vi "COBS_Unstuff.vi"(8 "error in (no error)":errorcluster, 11 "Suffed data":string) -> (0 "error out":errorcluster, 2 "Valid?":bool, 3 "Unstuffed String":string)   [LabVIEW 2015, in "Shore Library.lvlib"]
doc: "Unstuffs data stuffed with the COBS algorithm. This is used to take zeros out of a byte array to allow it to be used as a delimeter. \n\nhttps://en.wikipedia.org/wiki/Consistent_Overhead_Byte_Stuffing"
uses:
  Shore Library.lvlib
panel:
  out "unsigned byte array":u8[](array[numeric])
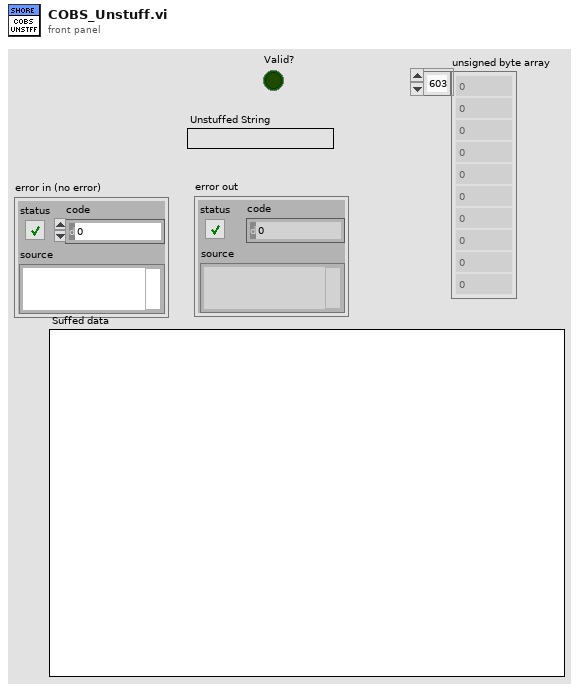
[diagram p1: front panel]
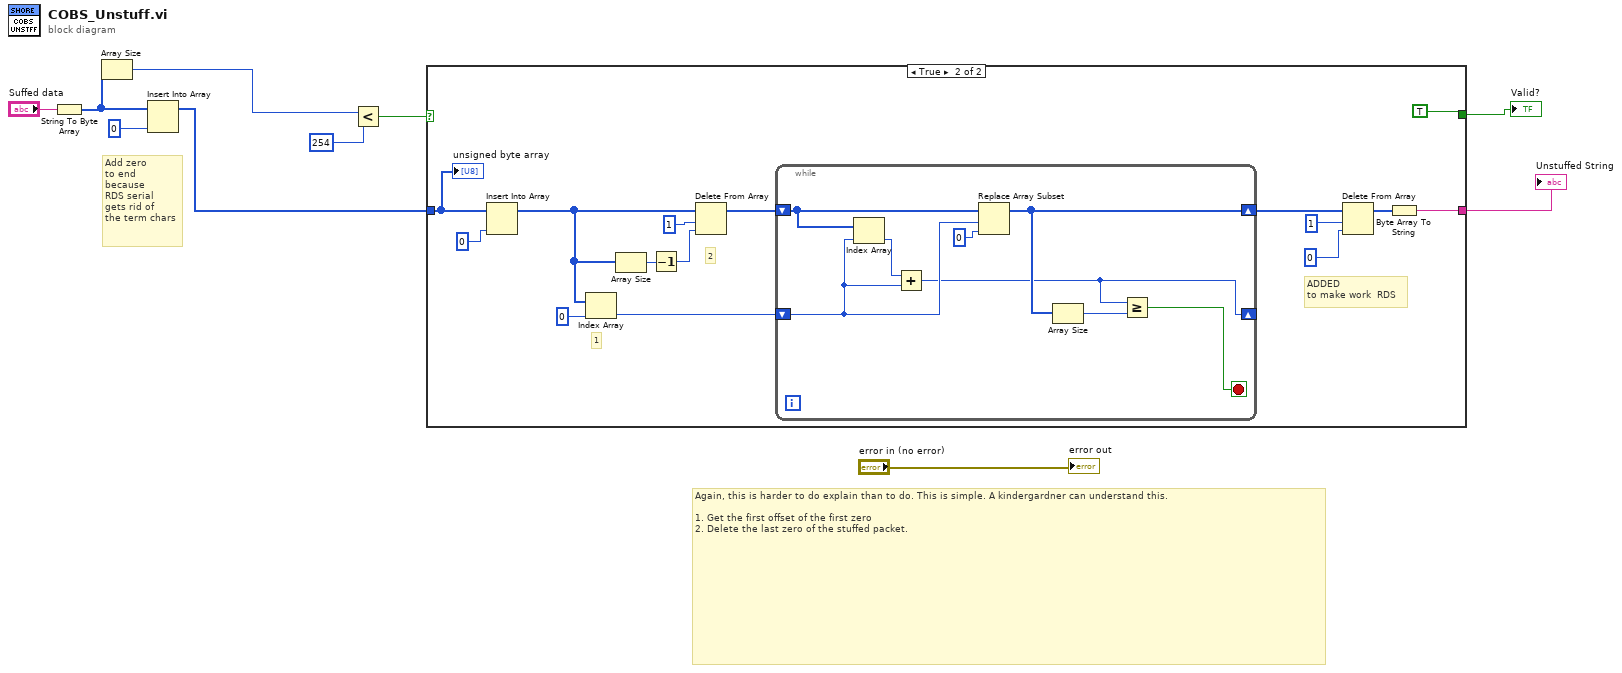
[diagram p0: block diagram]
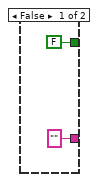
[diagram p2: hidden frame]
diagram:
  # "Add zero \nto end\nbecause \nRDS serial \ngets rid of \nthe term chars"
  # "Again, this is harder to do explain than to do. This is simple. A kindergardner can understand this. \n\n1. Get the first offset of the first zero\n2. Delete the last zero of the stuffed packet."
  n1 = String To Byte Array(string="Suffed data") -> (unsigned byte array=w2:u8[])
  n2 = Array Size(array=w2) -> (size(s)=w1:i32)
  n3 = Insert Into Array(array=w2, new element=u8 0) -> (w3:u8[])  [unwired: 1 in]
  n4 = Less?(x=w1, y=254) -> (x < y?=w5:bool)
  n5 = case shown="True" w5 {
    tunnel: ["" ("string") w15] -> w8
    tunnel: w3 -> [_ w14]
    tunnel: [FALSE TRUE] -> w6
    frame False {
    }
    frame True {
      # "ADDED\nto make work  RDS"
      # "2"
      # "1"
      n6 = Insert Into Array(array=w14, new element=u8 0 ("index")) -> (w17:u8[])  [unwired: 1 in]
      n7 = Index Array(array=w17, index=0) -> (element=w20:u8)
      n8 = Array Size(array=w17) -> (size(s)=w23:i32)
      n9 = Decrement(x=w23) -> (x-1=w24:i32)
      n10 = Delete From Array(array=w17, length=1, index=w24) -> (array with subset deleted=w21:u8[])  [unwired: 1 out]
      n11 = while {
        shift-right: [w29] -> _
        shift-left: w20 -> [w32]
        shift-right: [w31] -> w25
        shift-left: w21 -> [w35]
        stop <- w28 stop-if-true
        n12 = Index Array(array=w35, index=w32) -> (element=w33:u8)
        n13 = Add(x=w33, y=w32) -> (x+y=w29:u8)
        n14 = Replace Array Subset(array=w35, new element=u8 0 ("new element/subarray"), index=w32) -> (w31:u8[])
        n15 = Array Size(array=w31) -> (size(s)=w30:i32)
        n16 = Greater Or Equal?(x=w29, y=w30) -> (x >= y?=w28:bool)
      }
      n17 = Delete From Array(array=w25, length=1, index=0) -> (array with subset deleted=w16:u8[])  [unwired: 1 out]
      n18 = Byte Array To String(unsigned byte array=w16) -> (string=w15:string)
      "unsigned byte array" <- w14
    }
  }
  "Unstuffed String" <- w8
  "Valid?" <- w6
  "error out" <- "error in (no error)"
